vi "PowerAnalyser.vi"() -> ()   [LabVIEW 2013]
uses:
  <vilib>/measure/maspectr.llb/Power Spectrum and PSD Export Mode.ctl
  <vilib>/Analysis/4window.llb/windowTd.ctl
  <vilib>/DAQmx/read.llb/DAQmx Read (Analog 2D DBL NChan NSamp).vi
  <vilib>/Analysis/baseanly.llb/Mean (DBL).vi
  <vilib>/DAQmx/create/channels.llb/DAQmx Create Channel (AI-Voltage-Basic).vi
  <vilib>/DAQmx/configure/timing.llb/DAQmx Timing (Sample Clock).vi
  <vilib>/measure/maspectr.llb/FFT Power Spectrum and PSD for 1 Chan.vi
  <vilib>/DAQmx/miscellaneous.llb/DAQmx Fill In Error Info.vi
  <vilib>/Analysis/NI_AALBase.lvlib
  <vilib>/measure/NI_MAPro.lvlib
  <vilib>/Analysis/NI_AALPro.lvlib
panel:
  in  "?":enum32{""}(tab)
  out "code":i32
  out "status":bool
  out "DAQ LOGs":string
  in  "?":bool
  out "Ticks":i32
  out "?":errorcluster
  out "Capacitive/Inductive":bool
  in  "?":enum32{"Hardware", "Software", "Help"}(tab)
  in  "?":T1(tab)
  in  "physical channels":tag
  in  "timeout":dbl=10.0 format="%0.2f"
  in  "input terminal configuration":i32(ring)=-1 items=["Default"=-1, "RSE"=10083, "NRSE"=10078, "Differential"=10106, "Pseudodifferential"=12529]
  in  "maximum value":dbl=5.0 format="%0.2f"
  in  "minimum value":dbl=-5.0 format="%0.2f"
  in  "sample mode":i32(ring)=10178 items=["Finite Samples"=10178, "Continuous Samples"=10123, "Hardware Timed Single Point"=12522]
  in  "rate":dbl=1000.0 format="%0.2f"
  in  "samples per channel":i32=1000
  in  "number of samples per channel":i32=-1
  out "Voltage":dbl[](graph) caption="MQ-135"
  out "Current":dbl[](graph)
  out "Current Scaled":dbl[](graph) caption="MQ-135"
  out "Voltage Scaled":dbl[](graph) caption="MQ-135"
  in  "?":enum32{"RMS", "Power 1", "Power 2", "FFT"}(tab)
  out "I RMS":dbl(graph) caption="MQ-135"
  out "Voltage RMS":dbl(graph) caption="MQ-135"
  out "Value":dbl
  out "Instant Real Power - P(W)":dbl[](graph) caption="MQ-135"
  out "Power Factor PF":dbl(graph) caption="MQ-135"
  out "Real Power - P(W)":dbl(graph) caption="MQ-135"
  out "Reactive Power (Q)":dbl(graph) caption="MQ-135"
  out "Apparent Power S (VA)":dbl(graph) caption="MQ-135"
  out "FFT Graph":cluster{"f0":dbl, "df":dbl, "magnitude":dbl[]}(graph)
  in  "export mode":T2 items=["Power Spectrum", "Power Spectral Density"]
  out "Power Spectrum / PSD":cluster{"f0":dbl, "df":dbl, "magnitude":dbl[]} {"magnitude" format="%.2p"; "f0" format="%0.2p"; "df" format="%0.2p"}
  in  "dB On (F)":bool
  in  "averaging (F)":bool
  in  "window":T3=1 items=["Rectangle"=0, "Hanning"=1, "Hamming"=2, "Blackman-Harris"=3, "Exact Blackman"=4, "Blackman"=5, "Flat Top"=6, "4 Term B-Harris "=7, "7 Term B-Harris"=8, "Low Sidelobe"=9, "Blackman Nuttall"=11, "Triangle"=30, "Bartlett-Hanning"=31, "Bohman"=32, "Parzen"=33, "Welch"=34, "Kaiser"=60, "Dolph-Chebyshev"=61, "Gaussian"=62]
  in  "file path":path
  in  "Save Button":bool
  # "Power Analyser V1.0"
  # "Dev1/ai0,Dev1/ai1"
  # "PWM_SIG"
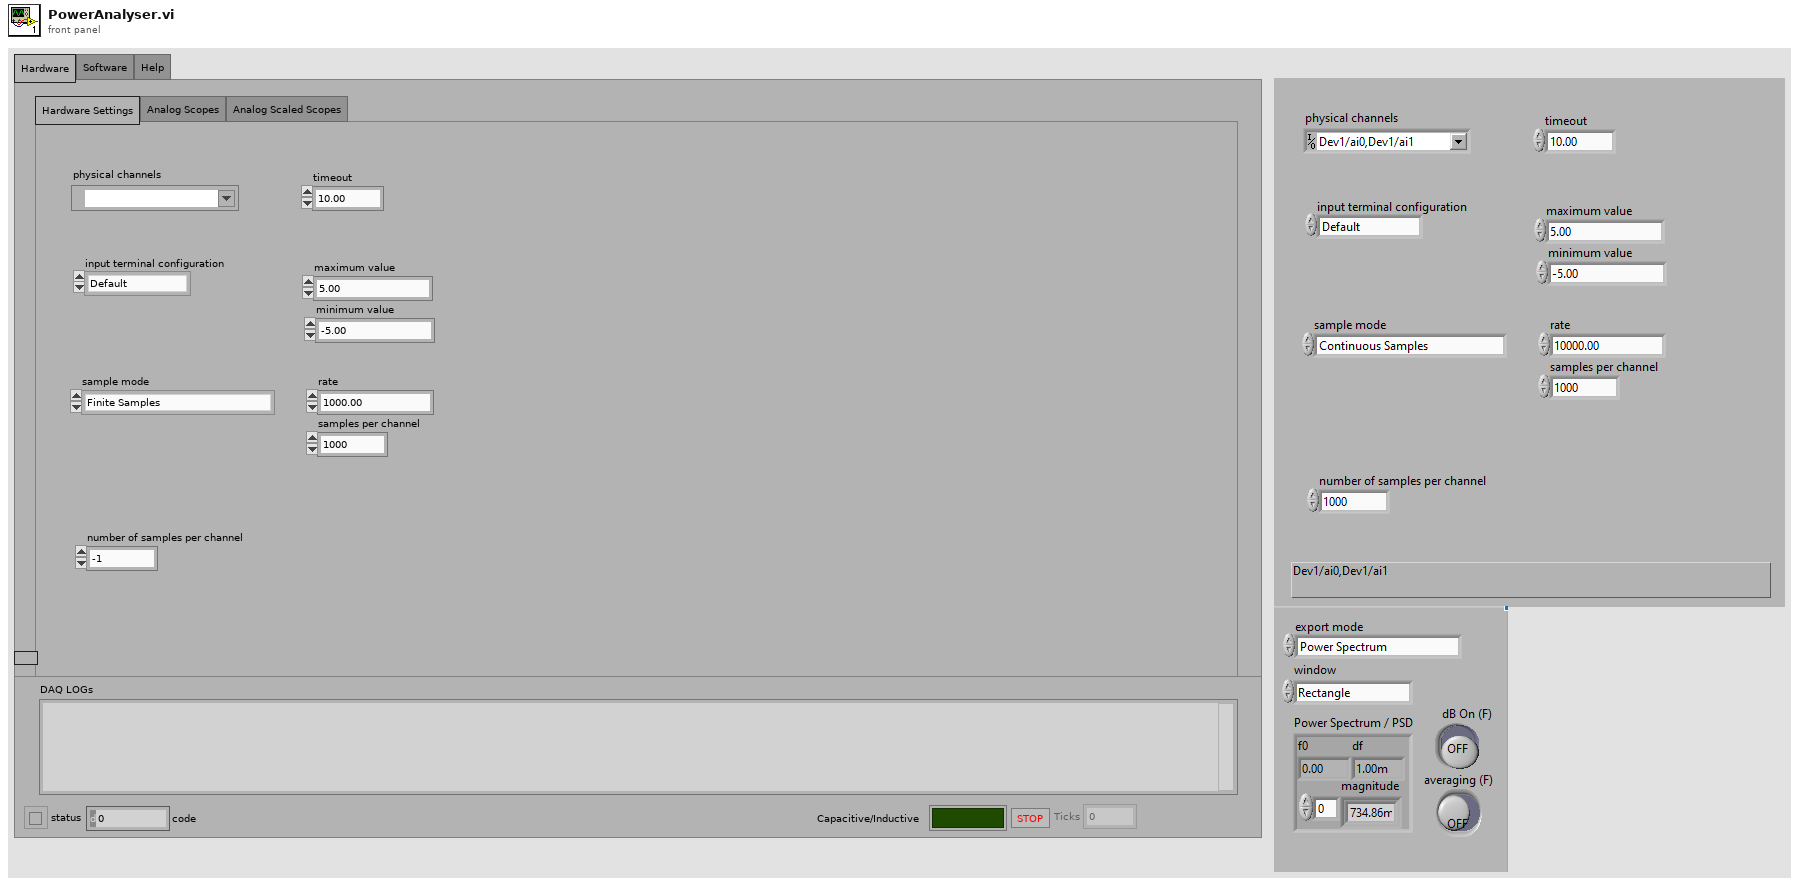
[diagram p1: front panel]
types:
  T1 = enum32{"Hardware Settings", "Analog Scopes", "Analog Scaled Scopes"}
  T2 = typedef "NI_MAPro.lvlib/Power Spectrum and PSD Export Mode.ctl" = u16
  T3 = typedef "NI_AALPro.lvlib/windowTd.ctl" = u32
  T4 = enum16{"open", "replace", "create", "open or create", "replace or create", "replace or create with confirmation"}
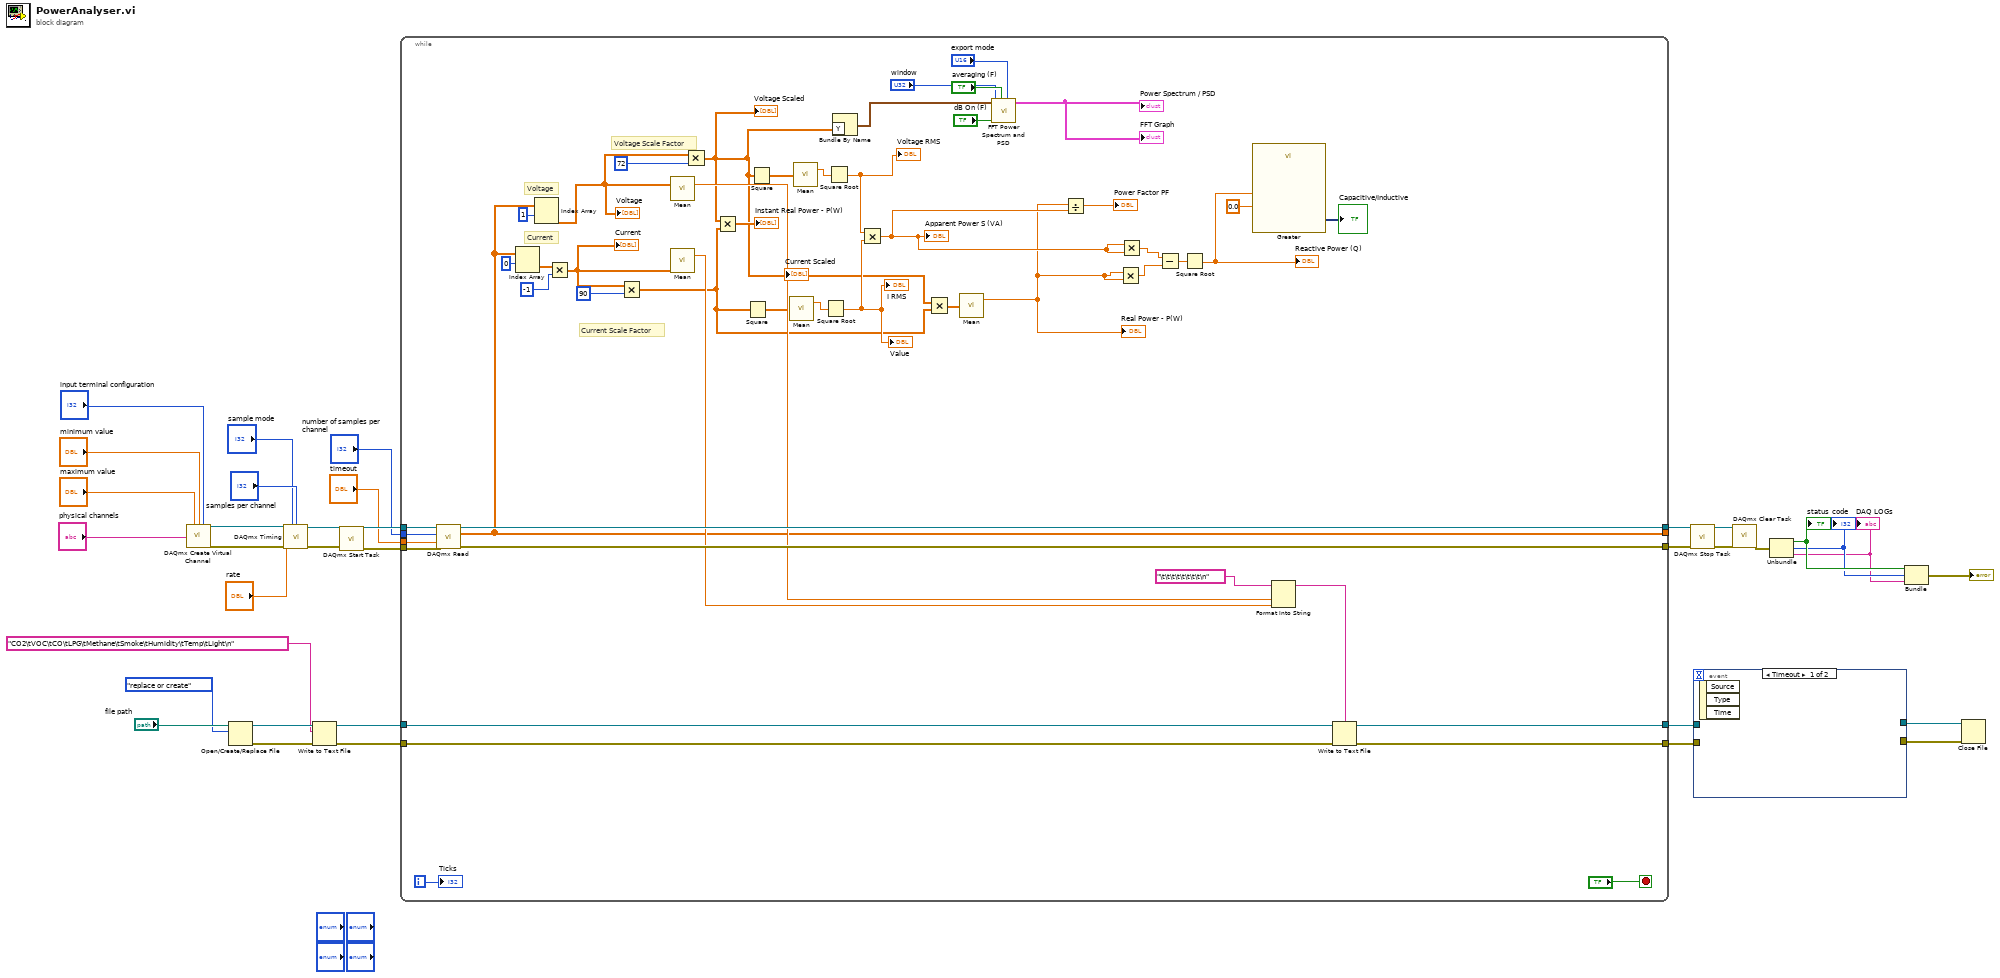
[diagram p0: block diagram]
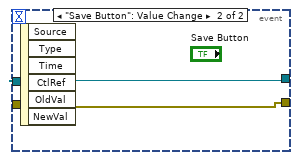
[diagram p2: hidden frame]
diagram:
  n1 = call-poly <vilib>:"DAQmx Create Virtual Channel.vi"("maximum value"="maximum value", "minimum value"="minimum value", "input terminal configuration"="input terminal configuration", "physical channels"="physical channels") -> ("task out"=w31:refnum<k21>, "error out"=w30:errorcluster)  [unwired: 10 in]
  n2 = Open/Create/Replace File(file path (use dialog)="file path", operation (0:open)=T4."replace or create") -> (refnum out=w5:refnum<file>, error out=w4:errorcluster)  [unwired: 4 in, 1 out]
  n3 = call-poly <vilib>:"DAQmx Timing.vi"("task/channels in"=w31, "sample mode"="sample mode", "samples per channel"="samples per channel", "rate"="rate", "error in"=w30) -> ("task out"=w26:refnum<k21>, "error out"=w25:errorcluster)  [unwired: 9 in]
  n4 = Write to Text File(file (use dialog)=w5, text="CO2\tVOC\tCO\tLPG\tMethane\tSmoke\tHumidity\tTemp\tLight\n", error in=w4) -> (refnum out=w3:refnum<file>, error out=w2:errorcluster)  [unwired: 1 in, 1 out]
  n5 = call <vilib>:"DAQmx Start Task.vi"("task/channels in"=w26, "error in"=w25) -> ("task out"=w24:refnum<k21>, "error out"=w23:errorcluster)  [unwired: 12 in]
  n6 = while {
    tunnel: w24 -> [w85]
    tunnel: w23 -> [w84]
    tunnel: "timeout" -> [w83]
    tunnel: [w82] -> w18
    tunnel: [w81] -> w17
    tunnel: [w56] -> _
    tunnel: "number of samples per channel" -> [w78]
    tunnel: w3 -> [w75]
    tunnel: w2 -> [w74]
    tunnel: [w72] -> w8
    tunnel: [w71] -> w6
    i -> [w76]
    stop <- "?" stop-if-true
    # "Current Scale Factor"
    # "Voltage Scale Factor"
    # "Current"
    # "Voltage"
    n7 = call-poly <vilib>:"DAQmx Read.vi"("task/channels in"=w85, "number of samples per channel"=w78, "timeout"=w83, "error in"=w84) -> ("task out"=w82:refnum<k21>, "data"=w56:dbl[][], "error out"=w81:errorcluster)  [unwired: 9 in]
    n8 = Index Array(array=w56, index (row)=0 ("index")) -> (element=w42:dbl[])  [unwired: 1 in]
    n9 = Index Array(array=w56, index (row)=1 ("index")) -> (element=w65:dbl[])  [unwired: 1 in]
    "Voltage" <- w65
    n10 = Multiply(x=w42, y=-1 ("index")) -> (x*y=w43:dbl[])
    "Current" <- w43
    n11 = Multiply(x=w43, y=90) -> (x*y=w46:dbl[])
    n12 = call-poly <vilib>:"Mean.vi"("X"=w65) -> ("mean"=w70:dbl)  [unwired: 1 out]
    n13 = call-poly <vilib>:"Mean.vi"("X"=w43) -> ("mean"=w69:dbl)  [unwired: 1 out]
    n14 = Multiply(x=w65, y=72) -> (x*y=w40:dbl[])
    "Voltage Scaled" <- w40
    n15 = Multiply(x=w40, y=w46) -> (x*y=→"Instant Real Power - P(W)":dbl[])
    n16 = Square(x=w46) -> (x^2=w62:dbl[])
    n17 = Square(x=w40) -> (x^2=w64:dbl[])
    n18 = call-poly <vilib>:"Mean.vi"("X"=w62) -> ("mean"=w61:dbl)  [unwired: 1 out]
    n19 = call-poly <vilib>:"Mean.vi"("X"=w64) -> ("mean"=w63:dbl)  [unwired: 1 out]
    n20 = Square Root(x=w61) -> (sqrt(x)=w47:dbl)
    "I RMS" <- w47
    "Value" <- w47
    n21 = Square Root(x=w63) -> (sqrt(x)=w48:dbl)
    "Voltage RMS" <- w48
    n22 = Bundle By Name("Y"=w40) -> (w51:waveform(dbl))  [unwired: 1 in]
    n23 = Multiply(x=w48, y=w47) -> (x*y=w39:dbl)
    "Apparent Power S (VA)" <- w39
    n24 = Multiply(x=w40, y=w46) -> (x*y=w45:dbl[])
    n25 = call-poly <vilib>:"Mean.vi"("X"=w45) -> ("mean"=w38:dbl)  [unwired: 1 out]
    "Real Power - P(W)" <- w38
    n26 = call-poly <vilib>:"FFT Power Spectrum and PSD.vi"("export mode"="export mode", "restart averaging (F)"="averaging (F)", "dB On (F)"="dB On (F)", "window"="window", "time signal"=w51) -> ("Power Spectrum / PSD"=→"Power Spectrum / PSD" →"FFT Graph":cluster{"f0":dbl, "df":dbl, "magnitude":dbl[]})  [unwired: 3 in, 3 out]
    n27 = Divide(x=w38, y=w39) -> (x/y=→"Power Factor PF":dbl)
    n28 = Multiply(x=w38, y=w38) -> (x*y=w36:dbl)
    n29 = Multiply(x=w39, y=w39) -> (x*y=w37:dbl)
    n30 = Subtract(x=w37, y=w36) -> (x-y=w59:dbl)
    n31 = Square Root(x=w59) -> (sqrt(x)=w44:dbl)
    "Reactive Power (Q)" <- w44
    n32 = call "Greater"("Constant Value to Compare Against"=0.0, "Operand 1"=w44) -> ("Result"=→"Capacitive/Inductive":dynamicdata)  [unwired: 8 in, 1 out]
    n33 = Format Into String(initial string="\t\t\t\t\t\t\t\t\n" ("format string"), w70, w69) -> (resulting string=w73:string)  [unwired: 2 in, 1 out]
    n34 = Write to Text File(file (use dialog)=w75, text=w73, error in=w74) -> (refnum out=w72:refnum<file>, error out=w71:errorcluster)  [unwired: 1 in, 1 out]
    "Ticks" <- w76
  }
  n35 = call <vilib>:"DAQmx Stop Task.vi"("task/channels in"=w18, "error in"=w17) -> ("task out"=w20:refnum<k21>, "error out"=w19:errorcluster)  [unwired: 12 in]
  n36 = event shown="[0] Timeout" {
    selector: _ -> [_ _]
    dyn-events: _ -> [_ _]
    timeout: _ -> [_ _]
    tunnel: [_ w87] -> w9
    tunnel: w8 -> [_ w87]
    tunnel: [_ w86] -> w7
    tunnel: w6 -> [_ w86]
    event Timeout {
      n37 = event-data() -> ()  [unwired: 1 in, 3 out]
    }
    event "Save Button": Value Change {
      n38 = event-data() -> ()  [unwired: 1 in, 6 out]
    }
  }
  n39 = call <vilib>:"DAQmx Clear Task.vi"("task in"=w20, "error in"=w19) -> ("error out"=w16:errorcluster)  [unwired: 13 in]
  n40 = Unbundle(w16) -> ("status"=w15:bool, "code"=w14:i32, "source"=w13:string)
  "DAQ LOGs" <- w13
  "status" <- w15
  "code" <- w14
  n41 = Bundle("status"=w15, "code"=w14, "source"=w13) -> (→"?":errorcluster)  [unwired: 1 in]
  n42 = Close File(refnum=w9, error in=w7) -> ()  [unwired: 2 out]
